vi "SPI_CRC.vi"(0 "Message":u8[](array[numeric]) format="%.0x") -> (1 "Message with CRC":u8[](array[numeric]), 2 "CRC":u8)   [LabVIEW 2015, in "navX-MXP IMU.lvlib"]
uses:
  navX-MXP IMU.lvlib
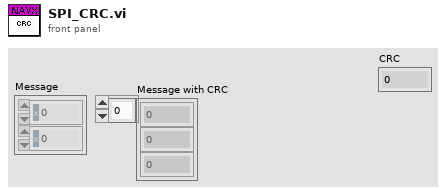
[diagram p1: front panel]
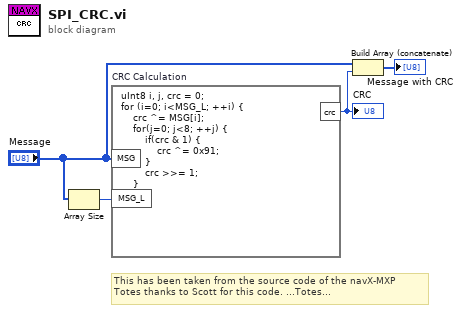
[diagram p0: block diagram]
diagram:
  # "This has been taken from the source code of the navX-MXP\nTotes thanks to Scott for this code. ...Totes..."
  n1 = Array Size(array="Message") -> (size(s)=w1:i32)
  n2 = formula code="uInt8 i, j, crc = 0;\nfor (i=0; i<MSG_L; ++i) {\n    crc ^= MSG[i];\n    for(j=0; j<8; ++j) {\n        if(crc & 1) {\n            crc ^= 0x91;\n        }\n        crc >>= 1;\n    }\n}" "CRC Calculation"("MSG"="Message", "MSG_L"=w1) -> ("crc"=w2:u8)
  "CRC" <- w2
  n3 = Build Array (concatenate)("Message", w2) -> (→"Message with CRC":u8[])
